vi "Coords Within Edge Range.vi"(10 "Horizontal":i32, 11 "Numeric":i32) -> (3 "Boolean":bool)   [LabVIEW 2015, in "LV Image Editor Framework.lvlib" / "Shape.lvclass"]
uses:
  Shape.lvclass
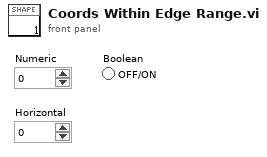
[diagram p1: front panel]
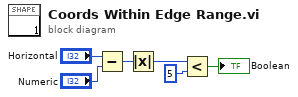
[diagram p0: block diagram]
diagram:
  n1 = Subtract(x="Horizontal", y="Numeric") -> (x-y=w2:i32)
  n2 = Absolute Value(x=w2) -> (abs(x)=w3:i32)
  n3 = Less?(x=w3, y=5) -> (x < y?=→"Boolean":bool)
